vi "2Dgauss.vi"(3 "output control":T1, 4 "data":variant, 5 "X":dbl[](array[numeric]), 6 "Coefficients":dbl[](array[numeric])) -> (0 "error out":errorcluster, 1 "f'(X,a)":dbl[][](array[numeric]), 2 "f(X,a)":dbl[](array[numeric]))   [LabVIEW 2014]
uses:
  <vilib>/gmath/NumericalOptimization/LM_output select.ctl
  <vilib>/gmath/NI_Gmath.lvlib
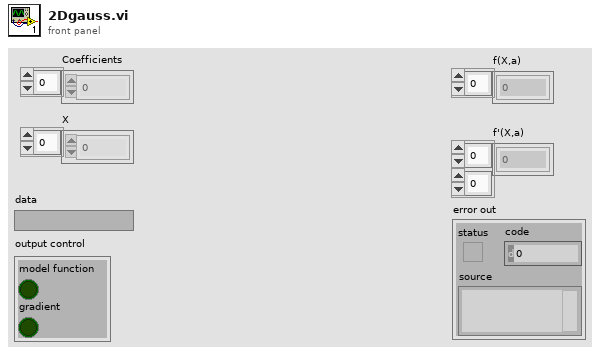
[diagram p1: front panel]
types:
  T1 = typedef "NI_Gmath.lvlib/LM_output select.ctl" = cluster{"model function":bool, "gradient":bool}
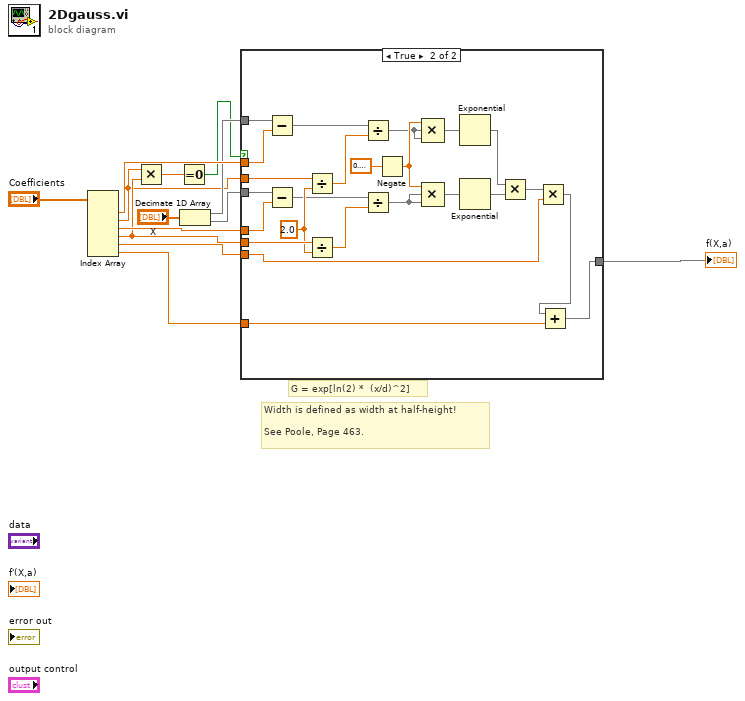
[diagram p0: block diagram]
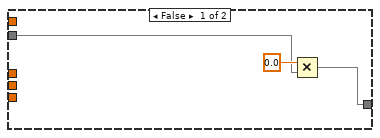
[diagram p2: hidden frame]
diagram:
  # "G = exp[ln(2) *  (x/d)^2]"
  # "Width is defined as width at half-height!\n\nSee Poole, Page 463."
  n1 = Index Array(array="Coefficients") -> (element #1=w13:dbl, element #2=w6:dbl, element #3=w10:dbl, element #4=w9:dbl, element #5=w5:dbl, element #6=w1:dbl)  [unwired: 6 in]
  n2 = Multiply(x=w6, y=w9) -> (x*y=w8:dbl)
  n3 = Equal To 0?(x=w8) -> (x = 0?=w2:bool)
  n4 = Decimate 1D Array("X") -> (w12:dbl[], w11:dbl[])
  n5 = case shown="True" w2 {
    tunnel: w13 -> [_ w40]
    tunnel: w12 -> [_ w39]
    tunnel: w11 -> [w14 w38]
    tunnel: w10 -> [_ w37]
    tunnel: w9 -> [_ w36]
    tunnel: w6 -> [_ w35]
    tunnel: w5 -> [_ w34]
    tunnel: [w16 w17] -> w3
    tunnel: w1 -> [_ w18]
    frame False {
      n6 = Multiply(x=0.0, y=w14) -> (x*y=w16:dbl[])
    }
    frame True {
      w30 = 2.0 ("y")
      n7 = Subtract(x=w39, y=w40) -> (x-y=w25:dbl[])
      n8 = Subtract(x=w38, y=w37) -> (x-y=w24:dbl[])
      n9 = Divide(x=w35, y=w30) -> (x/y=w32:dbl)
      n10 = Divide(x=w36, y=w30) -> (x/y=w31:dbl)
      n11 = Divide(x=w25, y=w32) -> (x/y=w26:dbl[])
      n12 = Divide(x=w24, y=w31) -> (x/y=w23:dbl[])
      n13 = Negate(x=0.6931471805599453) -> (-x=w28:dbl)
      n14 = Compound Arithmetic op=MULTIPLY(w28, w26, w26) -> (w27:dbl[])
      n15 = Compound Arithmetic op=MULTIPLY(w28, w23, w23) -> (w22:dbl[])
      n16 = Exponential(1:w27) -> (0:w20:dbl[])
      n17 = Exponential(1:w22) -> (0:w21:dbl[])
      n18 = Multiply(x=w20, y=w21) -> (x*y=w33:dbl[])
      n19 = Multiply(x=w33, y=w34) -> (x*y=w19:dbl[])
      n20 = Add(x=w19, y=w18) -> (x+y=w17:dbl[])
    }
  }
  "f(X,a)" <- w3
